vi "Old Control Panel.vi"(8 "error in (no error)":errorcluster, 11 "Fake cryostat in":refnum<class "Cryostat.lvclass">) -> (0 "error out":errorcluster, 3 "Fake cryostat out":refnum<class "Cryostat.lvclass">)   [LabVIEW 2017, in "Cryostat.lvclass"]
doc: "(Dynamic) A user-level application that simulates the physical front panel of the Instrument. Provide the user with buttons to manually control features of the instrument, and provide indicators of its current state."
uses:
  Cryostat.lvclass
  Cryostat.lvclass/Cryostat.ctl
  Utility Classes/Readable/Readable.lvclass
panel:
  out "In control mode?\n(not currently working)":bool
  in  "stop":bool
  in  "Set":bool
  in  "Read to Control":bool
  in  "Read":bool
  in  "Copy actual to set":bool
  in  "Populate fields with member data":bool
  out "Current set point":dbl
  in  "Desired set point":dbl
  out "Temperature B":dbl
  out "Temperature A":dbl
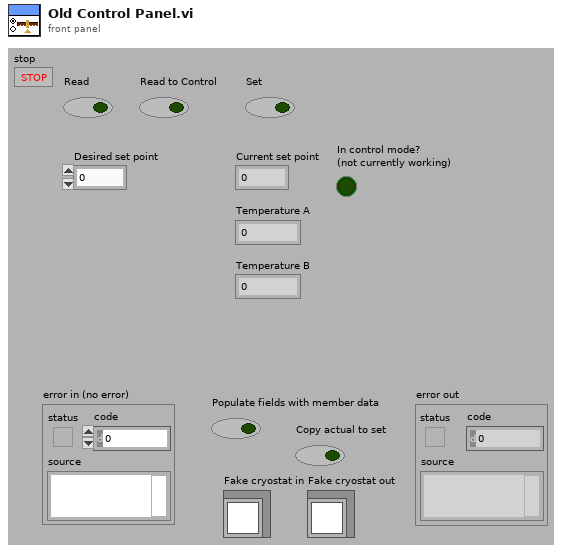
[diagram p1: front panel]
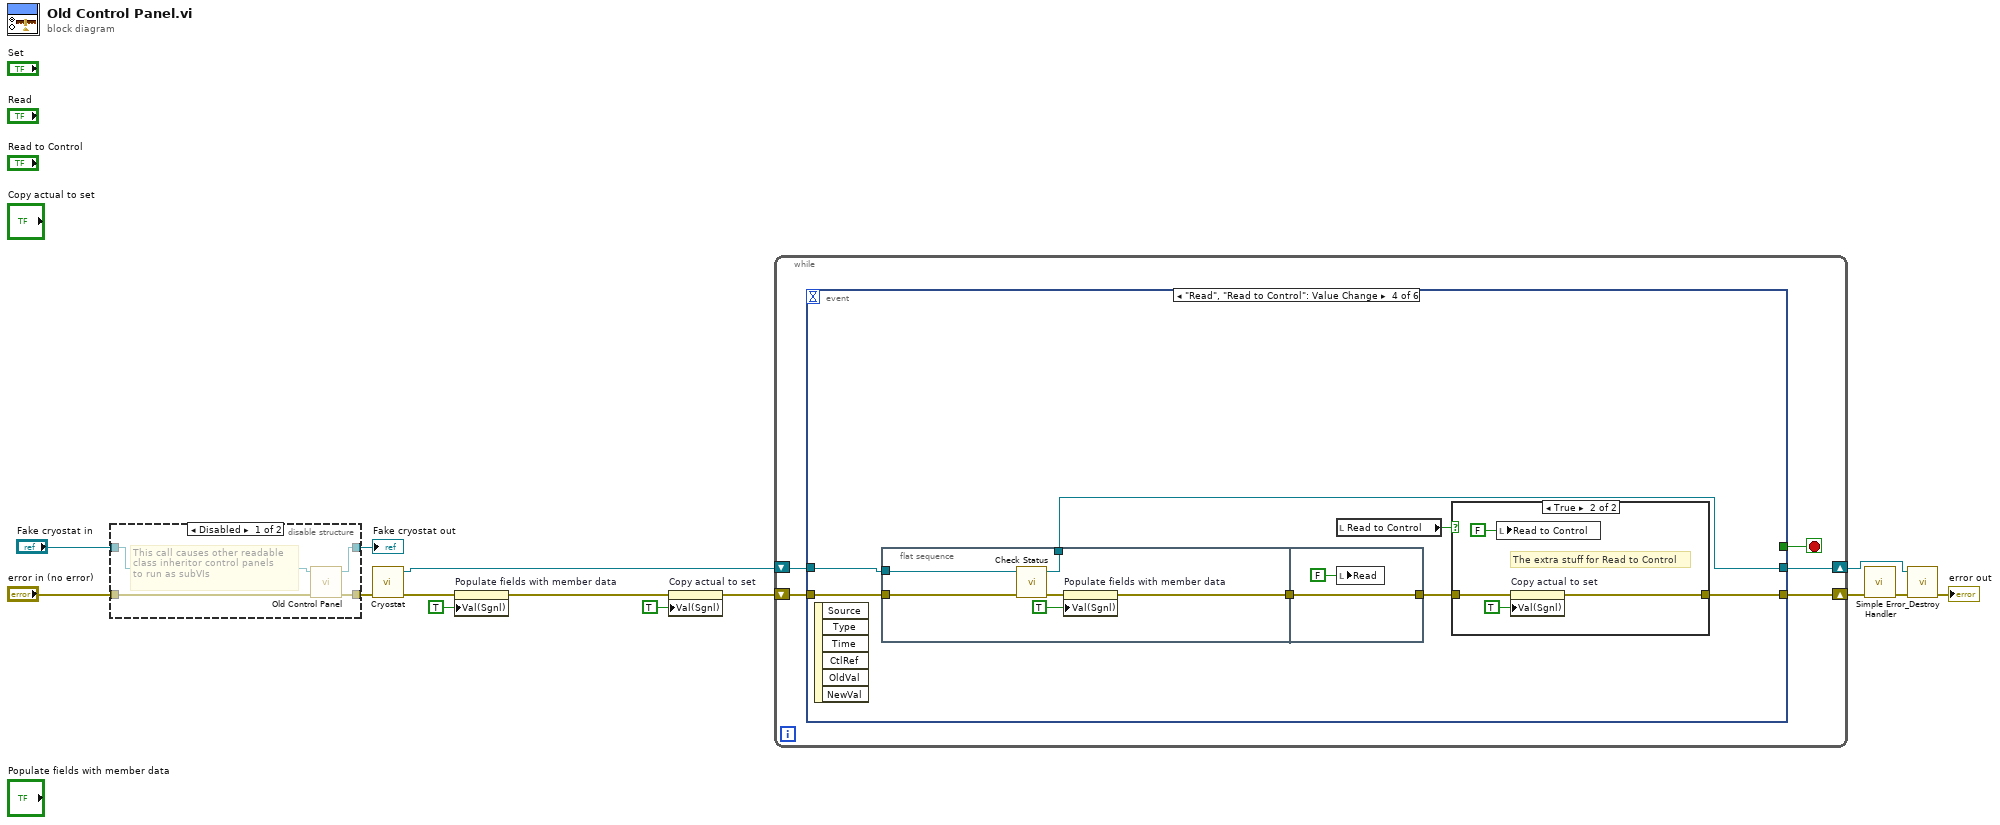
[diagram p0: block diagram]
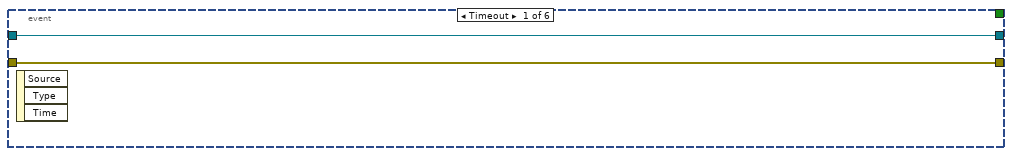
[diagram p3: hidden frame]
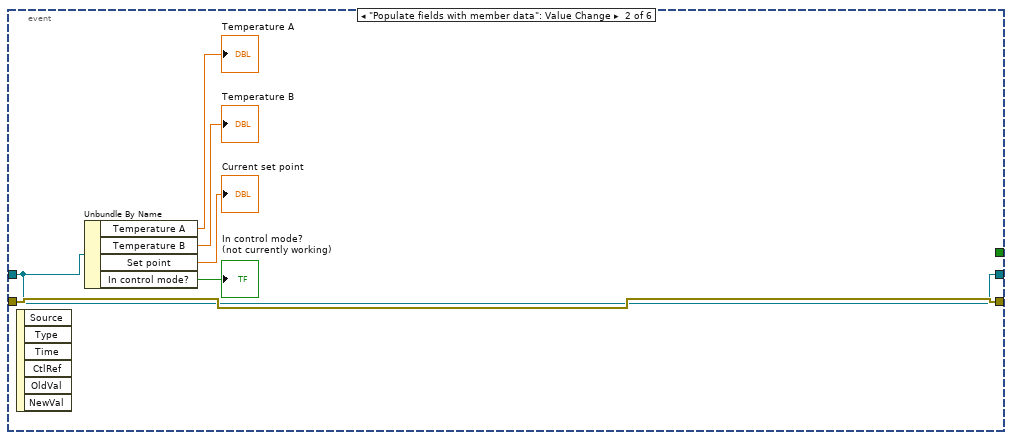
[diagram p4: hidden frame]
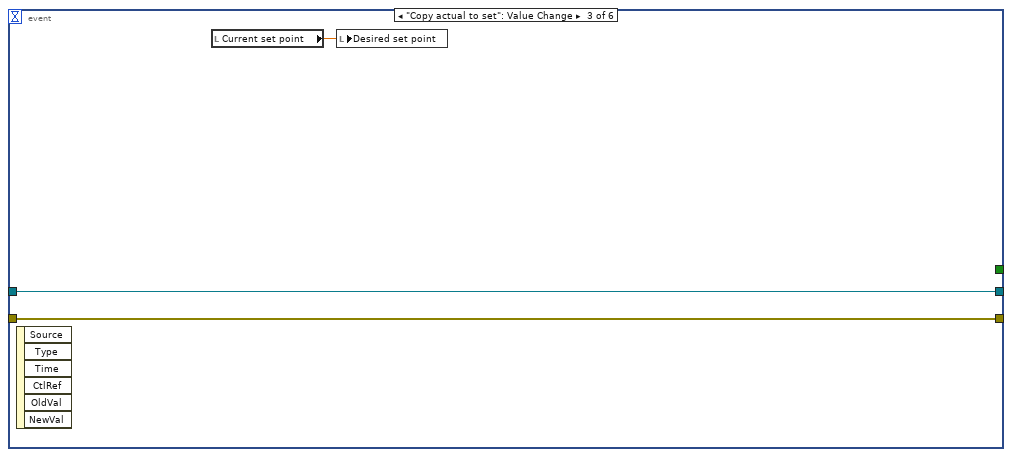
[diagram p5: hidden frame]
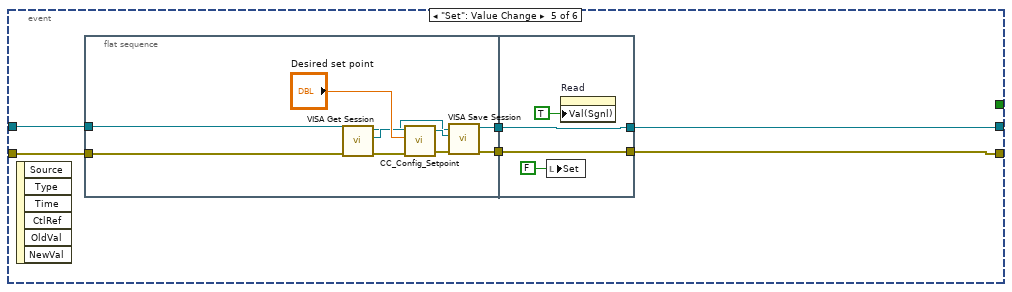
[diagram p7: hidden frame]
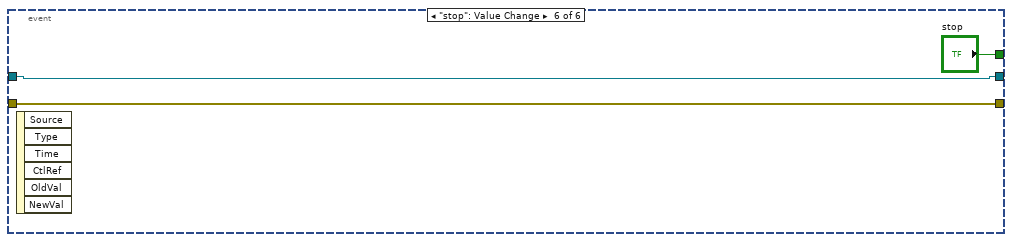
[diagram p8: hidden frame]
diagram:
  n1 = disable-structure shown="Disabled" {
    disable-tunnel: [w18 w20] -> w13
    disable-tunnel: "error in (no error)" -> [w17 w19]
    disable-tunnel: "Fake cryostat in" -> [w16 w20]
    disable-tunnel: [w15 w19] -> w11
    frame Disabled {
      # "This call causes other readable\nclass inheritor control panels\nto run as subVIs"
      n2 = call-parent "Old Control Panel.vi"("error in (no error)"=w17, "Instrument in"=w16) -> ("error out"=w15:errorcluster, "Instrument out"=w18:refnum<class "Cryostat.lvclass">)  [unwired: 8 out]
    }
    frame Enabled {
    }
  }
  "Fake cryostat out" <- w13
  n3 = call "Cryostat.vi"("error in (no error)"=w11) -> ("error out"=w10:errorcluster, "Cryostat out"=w5:refnum<class "Cryostat.lvclass">)  [unwired: 9 in]
  n4 = property on="Populate fields with member data" class="Bool (strict)"(error in=w10, "Val(Sgnl)"=TRUE ("Value (Signaling)")) -> (error out=w7:errorcluster)  [unwired: 1 in, 1 out]
  n5 = property on="Copy actual to set" class="Bool (strict)"(error in=w7, "Val(Sgnl)"=TRUE ("Value (Signaling)")) -> (error out=w6:errorcluster)  [unwired: 1 in, 1 out]
  n6 = while {
    shift-right: [w23] -> w4
    shift-left: w6 -> [w22]
    shift-right: [w25] -> w1
    shift-left: w5 -> [w24]
    stop <- w21 stop-if-true
    n7 = event shown="[3] \"Read\", \"Read to Control\": Value Change" {
      selector: _ -> [_ _ _ _ _ _]
      dyn-events: _ -> [_ _ _ _ _ _]
      timeout: _ -> [_ _ _ _ _ _]
      tunnel: [w27 w32 w36 w37 w60 w78] -> w25
      tunnel: w24 -> [w27 w32 w36 w40 w61 w78]
      tunnel: [w26 w33 w35 w38 w59 w77] -> w23
      tunnel: w22 -> [w26 w33 w35 w39 w62 w77]
      tunnel: [_ _ _ _ _ "stop"] -> w21
      event Timeout {
        n8 = event-data() -> ()  [unwired: 1 in, 3 out]
      }
      event "Populate fields with member data": Value Change {
        n9 = event-data() -> ()  [unwired: 1 in, 6 out]
        n10 = Unbundle By Name(w32) -> ("Temperature A"=→"Temperature A":dbl, "Temperature B"=→"Temperature B":dbl, "Set point"=→"Current set point":dbl, "In control mode?"=→"In control mode?\n(not currently working)":bool)
      }
      event "Copy actual to set": Value Change {
        n11 = event-data() -> ()  [unwired: 1 in, 6 out]
        n12 = local read "Current set point"() -> (w34:dbl)
        n13 = local write "Desired set point"(w34) -> ()
      }
      event "Read", "Read to Control": Value Change {
        n14 = event-data() -> ()  [unwired: 1 in, 6 out]
        n15 = flat-sequence {
          tunnel: w39 -> [w54]
          tunnel: w40 -> [w53]
          tunnel: [w52] -> w37
          tunnel: [w49] -> w43
          tunnel: [w55] -> w41
          tunnel: w43 -> [w55]
          frame #0 {
            n16 = call-dynamic "Check Status.vi"("error in (no error)"=w54, "Cryostat in"=w53) -> ("error out"=w51:errorcluster, "Cryostat out"=w52:refnum<class "Cryostat.lvclass">)  [unwired: 8 out]
            n17 = property on="Populate fields with member data" class="Bool (strict)"(error in=w51, "Val(Sgnl)"=TRUE ("Value (Signaling)")) -> (error out=w49:errorcluster)  [unwired: 1 in, 1 out]
          }
          frame #1 {
            n18 = local write "Read"(FALSE ("Read")) -> ()
          }
        }
        n19 = local read "Read to Control"() -> (w42:bool)
        n20 = case shown="True" w42 {
          tunnel: w41 -> [w44 w46]
          tunnel: [w44 w45] -> w38
          frame False {
          }
          frame True {
            # "The extra stuff for Read to Control"
            n21 = local write "Read to Control"(FALSE ("Read to Control")) -> ()
            n22 = property on="Copy actual to set" class="Bool (strict)"(error in=w46, "Val(Sgnl)"=TRUE ("Value (Signaling)")) -> (error out=w45:errorcluster)  [unwired: 1 in, 1 out]
          }
        }
      }
      event "Set": Value Change {
        n23 = event-data() -> ()  [unwired: 1 in, 6 out]
        n24 = flat-sequence {
          tunnel: w62 -> [w72]
          tunnel: w61 -> [w68]
          tunnel: [w65] -> w58
          tunnel: [w64] -> w57
          tunnel: [w75] -> w59
          tunnel: [w76] -> w60
          tunnel: w58 -> [w76]
          tunnel: w57 -> [w75]
          frame #0 {
            n25 = call-dynamic "VISA Get Session.vi"("error in (no error)"=w72, "Instrument.lvclass in"=w68) -> ("error out"=w69:errorcluster, "VISA Resource Name"=w70:refnum<visa-resource-name>, "Instrument.lvclass out"=w63:refnum<class "Cryostat.lvclass">)  [unwired: 7 out]
            n26 = call "CC_Config_Setpoint.vi"("error in (no error)"=w69, "Set Point"="Desired set point", "VISA In"=w70) -> ("error out"=w67:errorcluster, "VISA Out"=w66:refnum<visa-resource-name>)  [unwired: 1 in, 1 out]
            n27 = call-dynamic "VISA Save Session.vi"("error in (no error)"=w67, "VISA Resource Name"=w66, "Instrument.lvclass in"=w63) -> ("error out"=w64:errorcluster, "Instrument.lvclass out"=w65:refnum<class "Cryostat.lvclass">)  [unwired: 7 out]
          }
          frame #1 {
            n28 = local write "Set"(FALSE ("Set")) -> ()
            n29 = property on="Read" class="Bool (strict)"("Val(Sgnl)"=TRUE ("Value (Signaling)")) -> ()  [unwired: 2 in, 2 out]
          }
        }
      }
      event "stop": Value Change {
        n30 = event-data() -> ()  [unwired: 1 in, 6 out]
      }
    }
  }
  n31 = call <vilib>:"Simple Error Handler.vi"("error in (no error)"=w4) -> ("error out"=w3:errorcluster)  [unwired: 1 in, 7 out]
  n32 = call-dynamic "_Destroy.vi"("error in (no error)"=w3, "Instrument in"=w1) -> ("error out"=→"error out":errorcluster)  [unwired: 9 out]
